vi "Remove.vi"(8 "error in (no error)":errorcluster, 11 "output in":refnum<class "Output.lvclass">) -> (0 "error out":errorcluster, 3 "output out":refnum<class "Output.lvclass">)   [LabVIEW 2015, in "Output.lvclass"]
uses:
  Output.lvclass
  Output.lvclass/Output.ctl
  <vilib>/ActorFramework/Message Enqueuer/Message Enqueuer.lvclass/Message Enqueuer.ctl
  <vilib>/ActorFramework/Message Enqueuer/Enqueue.vi
  <vilib>/ActorFramework/Message Priority Queue/Priority Enqueue.vi
  <vilib>/ActorFramework/Stop Msg/Stop Msg.lvclass
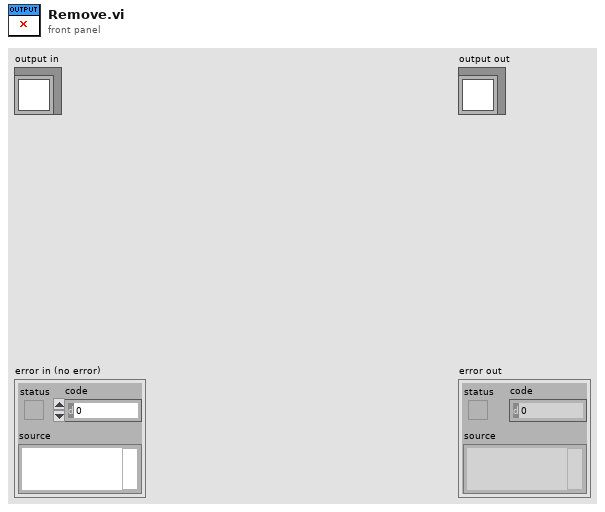
[diagram p1: front panel]
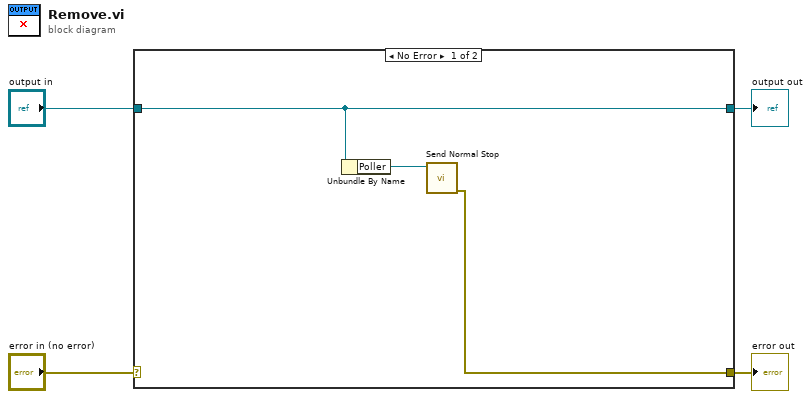
[diagram p0: block diagram]
diagram:
  n1 = case shown="No Error" "error in (no error)" {
    selector: "error in (no error)" -> [_ w9]
    tunnel: [w5 w9] -> w3
    tunnel: [w7 w8] -> w1
    tunnel: "output in" -> [w7 w8]
    frame No Error {
      n2 = Unbundle By Name(w7) -> ("Poller"=w6:refnum<class "Message Enqueuer.lvclass">)
      n3 = call <vilib>:"Send Normal Stop.vi"("Message Enqueuer"=w6) -> ("error out"=w5:errorcluster)  [unwired: 10 in]
    }
    frame Error {
    }
  }
  "error out" <- w3
  "output out" <- w1
